vi "Get Terminal Type.vi"(8 "error in":errorcluster, 11 "message or subaddress":T1 format="%.0x") -> (0 "error out":errorcluster, 2 "terminal type":enum16{"Bus Controller", "Remote Terminal"}(ring), 3 "message or subaddress out":T1 format="%.0x")   [LabVIEW 2020, in "AIM MIL-STD-1553 Scripting.lvlib"]
doc: "Returns the <b>terminal type</b> of the parent item where the <b>message or subaddress</b> is located. A message will return Bus Controller, and a subaddress will return Remote Terminal."
uses:
  AIM MIL-STD-1553 Scripting.lvlib
  <vilib>/NI VeriStand/Custom Device API/Custom Device Item Ref.ctl
  Constants.vi
  <vilib>/NI VeriStand/Custom Device API/Custom Device API.lvlib
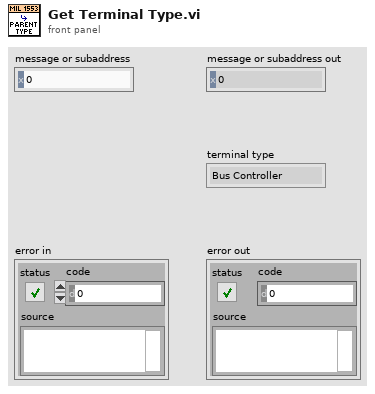
[diagram p1: front panel]
types:
  T1 = typedef "Custom Device API.lvlib/Custom Device Item Ref.ctl" = u64
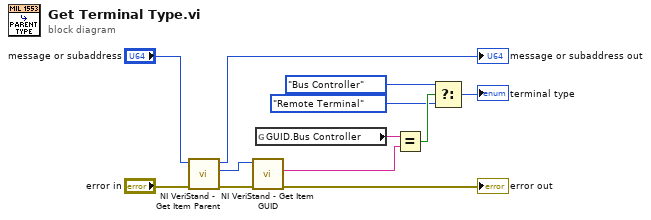
[diagram p0: block diagram]
diagram:
  n1 = call <vilib>:"NI VeriStand - Get Item Parent.vi"("error in (no error)"="error in", "Item Ref in"="message or subaddress") -> ("error out"=w8:errorcluster, "Parent Ref"=w9:T1, "Item Ref out"=→"message or subaddress out":T1)  [unwired: 6 in, 1 out]
  n2 = call <vilib>:"NI VeriStand - Get Item GUID.vi"("error in (no error)"=w8, "Item Ref in"=w9) -> ("error out"=→"error out":errorcluster, "GUID"=w6:string)  [unwired: 7 in, 1 out]
  n3 = global read "Constants.vi" "GUID.Bus Controller"() -> (w7:string)
  n4 = Equal?(x=w7, y=w6) -> (x = y?=w4:bool)
  n5 = Select(t=enum16{"Bus Controller", "Remote Terminal"}."Bus Controller", s=w4, f=enum16{"Bus Controller", "Remote Terminal"}."Remote Terminal") -> (s? t:f=→"terminal type":enum16{"Bus Controller", "Remote Terminal"})
